vi "Client - Simple.vi"(8 "error in (no error)":errorcluster, 9 "Data":variant, 10 "Command":string, 11 "RemoteControl in":refnum<class "RemoteControl.lvclass">) -> (0 "error out":errorcluster, 1 "Data out":variant, 2 "Command out":string, 3 "RemoteControl out":refnum<class "RemoteControl.lvclass">)   [LabVIEW 2016, in "RemoteControl.lvclass"]
uses:
  RemoteControl.lvclass
panel:
  in  "address":string
  out "# reads":i32
  out "execution time (ms)":u32
  # "Simple Client"
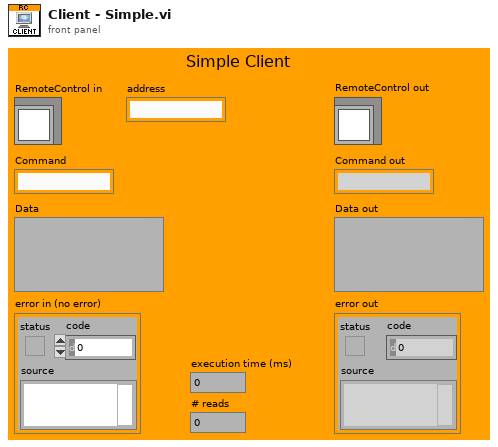
[diagram p1: front panel]
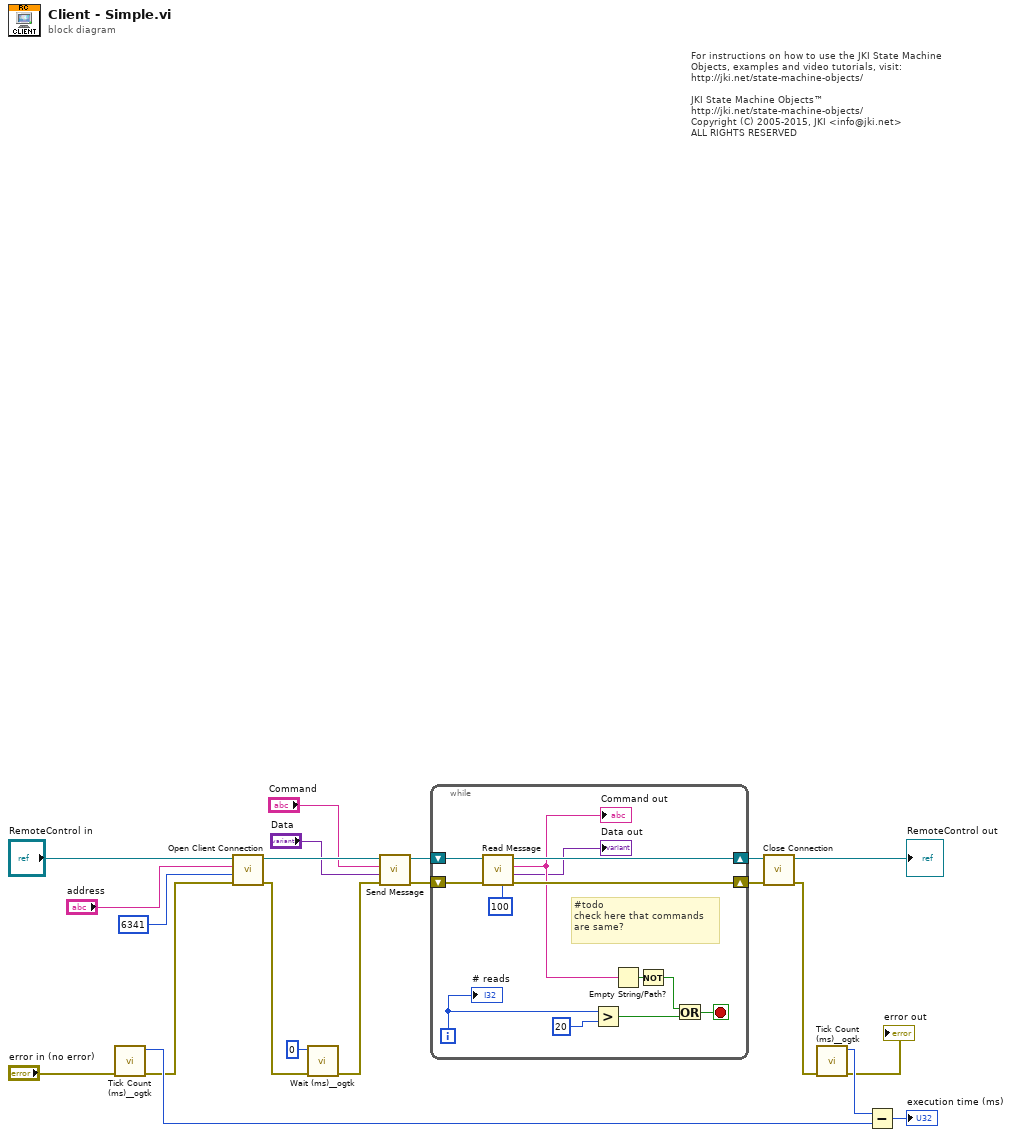
[diagram p0: block diagram]
diagram:
  # "For instructions on how to use the JKI State Machine Objects, examples and video tutorials, visit:\nhttp://jki.net/state-machine-objects/\n\nJKI State Machine Objects™\nhttp://jki.net/state-machine-objects/\nCopyright (C) 2005-2015, JKI <info@jki.net>\nALL RIGHTS RESERVED"
  n1 = call <userlib>:"Tick Count (ms)__ogtk.vi"("error in (no error)"="error in (no error)") -> ("error out"=w3:errorcluster, "millisecond timer value"=w18:u32)  [unwired: 9 in]
  n2 = call-dynamic "Open Client Connection.vi"("error in (no error)"=w3, "Port"=u32 6341, "address"="address", "RemoteControl in"="RemoteControl in") -> ("error out"=w9:errorcluster, "RemoteControl out"=w13:refnum<class "RemoteControl.lvclass">)  [unwired: 6 in]
  n3 = call <userlib>:"Wait (ms)__ogtk.vi"("error in (no error)"=w9, "milliseconds to wait"=u32 0) -> ("error out"=w10:errorcluster)  [unwired: 8 in, 1 out]
  n4 = call-dynamic "Send Message.vi"("error in (no error)"=w10, "Data"="Data", "Command"="Command", "RemoteControl in"=w13) -> ("error out"=w14:errorcluster, "RemoteControl out"=w15:refnum<class "RemoteControl.lvclass">)  [unwired: 6 in]
  n5 = while {
    shift-right: [w34] -> w17
    shift-left: w15 -> [w32]
    shift-right: [w33] -> w16
    shift-left: w14 -> [w31]
    i -> [w27]
    stop <- w28 stop-if-true
    # "#todo\ncheck here that commands\nare same?"
    n6 = call-dynamic "Read Message.vi"("timeout in ms (100)"=100, "error in (no error)"=w31, "RemoteControl in"=w32) -> ("error out"=w33:errorcluster, "Data"=→"Data out":variant, "Command"=w24:string, "RemoteControl out"=w34:refnum<class "RemoteControl.lvclass">)  [unwired: 4 in, 1 out]
    "Command out" <- w24
    n7 = Greater?(x=w27, y=20) -> (0:w26:bool)
    n8 = Empty String/Path?(string/path=w24) -> (empty?=w29:bool)
    n9 = Not(x=w29) -> (.not. x?=w22:bool)
    n10 = Or(x=w22, y=w26) -> (x .or. y?=w28:bool)
    "# reads" <- w27
  }
  n11 = call-dynamic "Close Connection.vi"("error in (no error)"=w16, "RemoteControl in"=w17) -> ("error out"=w8:errorcluster, "RemoteControl out"=→"RemoteControl out":refnum<class "RemoteControl.lvclass">)  [unwired: 8 in]
  n12 = call <userlib>:"Tick Count (ms)__ogtk.vi"("error in (no error)"=w8) -> ("error out"=→"error out":errorcluster, "millisecond timer value"=w21:u32)  [unwired: 9 in]
  n13 = Subtract(x=w21, y=w18) -> (x-y=→"execution time (ms)":u32)
